vi "XIPIN_UltraScale_FPGAs_Transceivers_Wizard_1_6.vi"   [LabVIEW 2017]
doc: "The UltraScale FPGAs Transceivers Wizard provides a simple and robust method of configuring one or more serial transceivers in UltraScale and UltraScale+ devices. Start from scratch, or use a configuration preset to target an industry standard. The highly flexible Transceivers Wizard generates a customized IP core for the transceivers, configuration options, and enabled ports you've selected, optionally including a variety of helper blocks to simplify common functionality. In addition, it can produce an example design for simple simulation and hardware usage demonstration.\n------------------------------------\n<b>Need License</b> : No"
uses:
  <vilib>/rvi/XilinxIP/XIPIN_XNode/niFpgaXIPIN.xnode
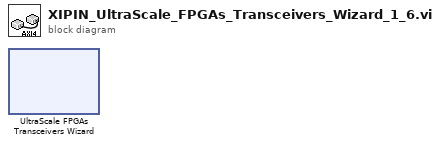
[diagram p0: block diagram]
diagram:
  n1 = xnode ("UltraScale FPGAs Transceivers Wizard")() -> ()
